vi "Calib_General_Setup.vi"(0 "Reference instrument":T3={"high limit (10V)"=4.0, "low limit (-10V)"=0.0, "Ch No"=4, "Off ch no"=0, "Calib filename"=path "", "Ref Instrument type"=enum."Enter Value"} {"Off ch no" min=0 max=1; "Ch No" min=0 max=7; "low limit (-10V)" min=-10 max=10 format="%.3f"; "high limit (10V)" min=-10 max=10 format="%.3f"}, 1 "Requested No of samples":i32=128 min=0 step=1, 2 "Sampling rate (Hz)":sgl=1000.0 format="%.2f", 5 "2nd ref instrument":T2={"2nd Ref type"=enum."LDA", "2nd inst present"=TRUE}, 9 "Temp":dbl=20.0 format="%.1f", 12 "Abs Press (mbar)":dbl=1005.0 format="%.2f") -> (8 "Output string":string, 10 "LDA Data":bool)   [LabVIEW 2017]
uses:
  Controls/Ref_Inst_type.ctl
  Controls/Graph_Type.ctl
  Globals/Meas_global.vi
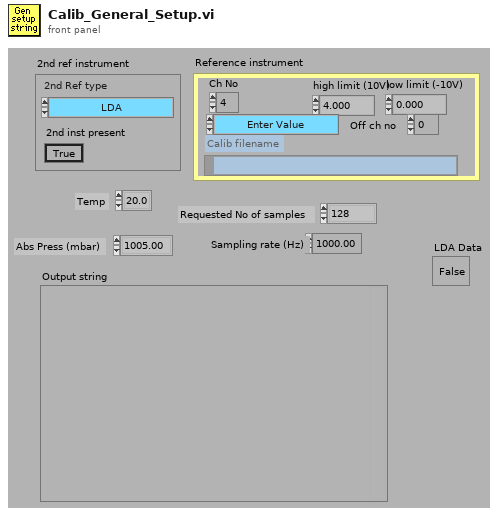
[diagram p1: front panel]
types:
  T1 = typedef "Ref_Inst_type.ctl" = enum16{"Propellor anemometer", "Pressure Transducer", "Raw voltage", "Pitot-static tube", "Preston tube", "Generic Linear", "Generic Polynomial", "Thermocouple", "LDA", "Enter Value", "ADAM Channel"}
  T2 = cluster{"2nd Ref type":T1, "2nd inst present":bool}
  T3 = cluster{"high limit (10V)":sgl, "low limit (-10V)":sgl, "Ch No":i16, "Off ch no":i8, "Calib filename":path, "Ref Instrument type":T1}
  T4 = typedef "Graph_Type.ctl" = enum16{"Show no graph", "Voltage trace", "Velocity trace", "Vel histogram", "Spectrum", "f.E(f) v Log f", "Auto-Corr"}
  T5 = cluster{"Plot 1":u16, "Plot 2":u16, "Save graph":u16, "Plot Type":T4}
  T6 = enum16{"From String to Cluster", "From Cluster to String"}
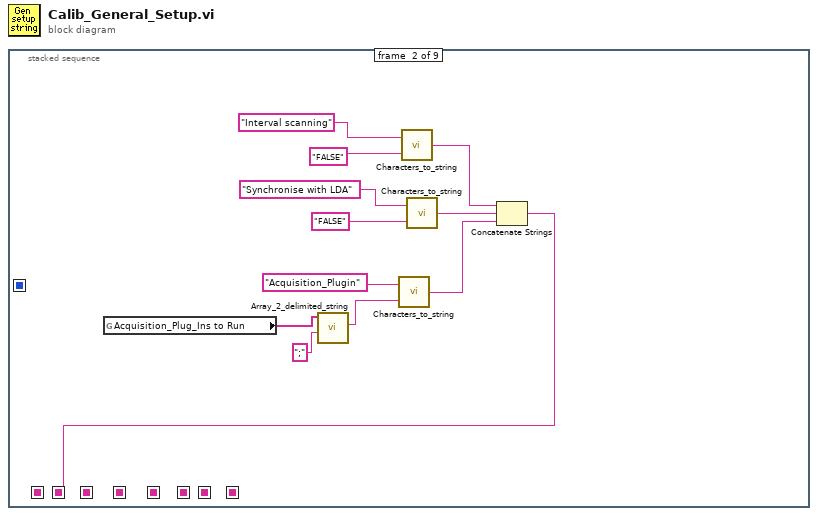
[diagram p0: block diagram]
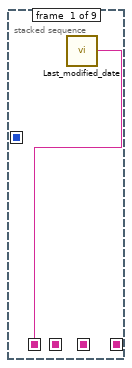
[diagram p2: hidden frame]
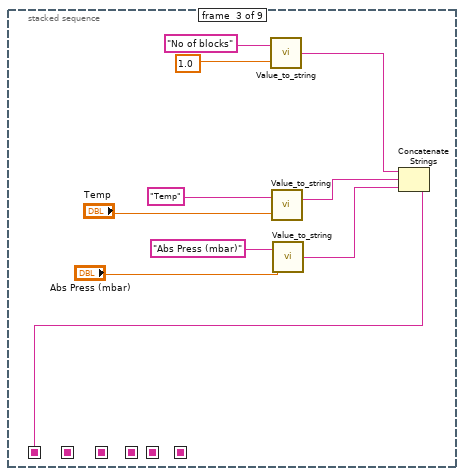
[diagram p3: hidden frame]
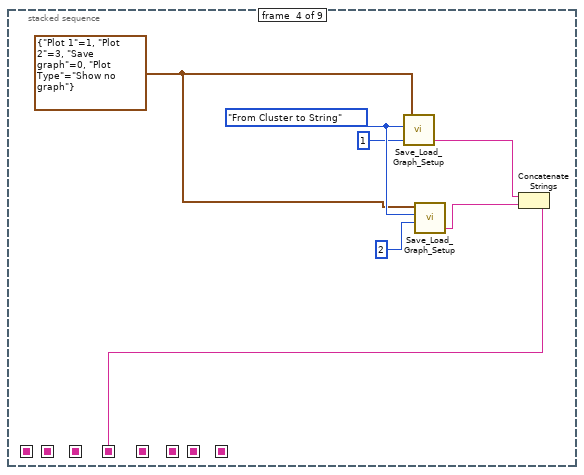
[diagram p4: hidden frame]
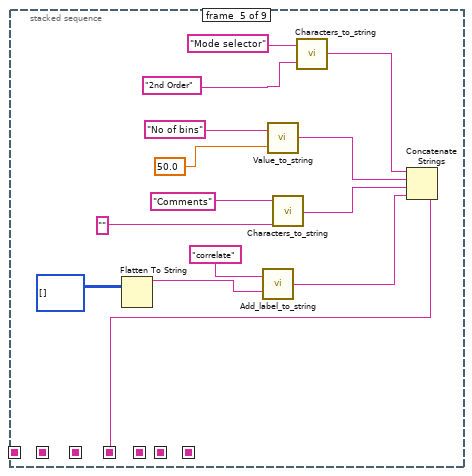
[diagram p5: hidden frame]
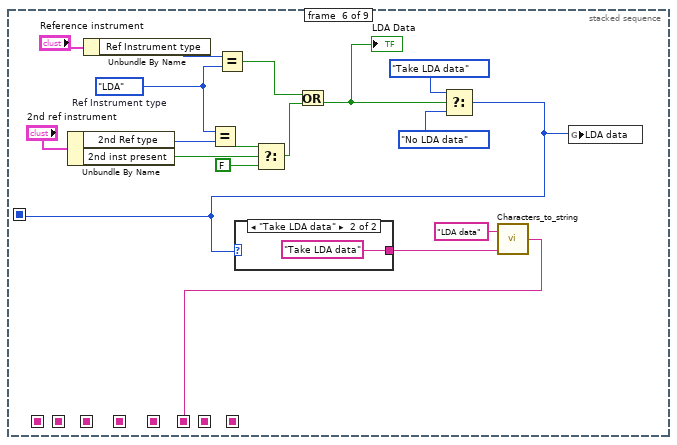
[diagram p6: hidden frame]
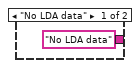
[diagram p7: hidden frame]
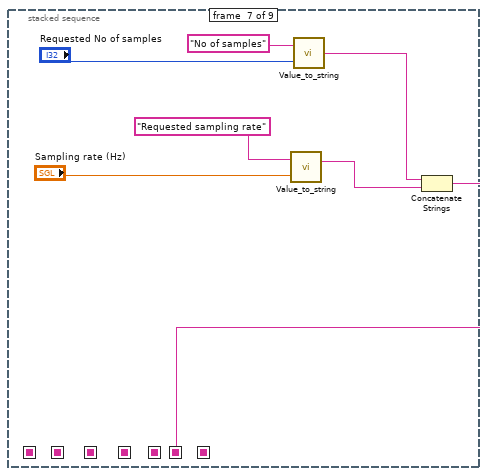
[diagram p8: hidden frame]
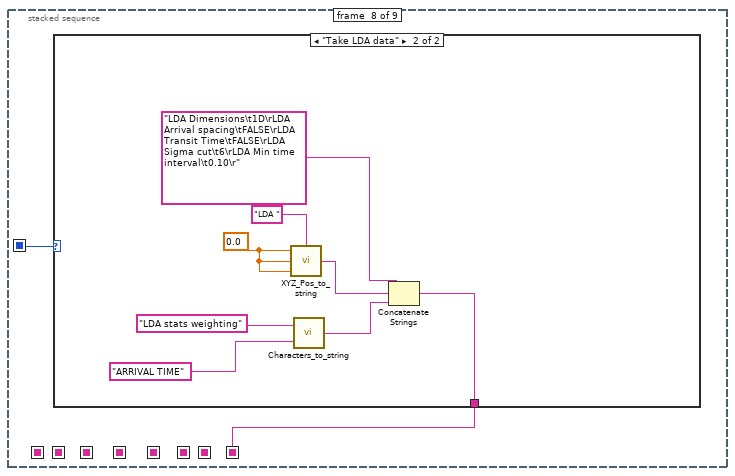
[diagram p9: hidden frame]
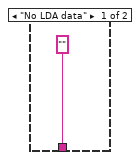
[diagram p10: hidden frame]
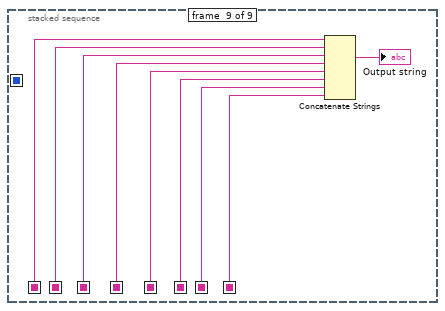
[diagram p11: hidden frame]
diagram:
  n1 = stacked-sequence {
    seq-local: [_ _ w22 _ _ _ _ _ _] -> [_ _ _ _ _ _ _ _ w90]
    seq-local: [_ w9 _ _ _ _ _ _ _] -> [_ _ _ _ _ _ _ _ w89]
    seq-local: [_ _ _ _ _ w59 _ _ _] -> [_ _ _ _ _ _ _ _ w85]
    seq-local: [_ _ _ _ _ _ w69 _ _] -> [_ _ _ _ _ _ _ _ w84]
    seq-local: [_ _ _ w25 _ _ _ _ _] -> [_ _ _ _ _ _ _ _ w87]
    seq-local: [_ _ _ _ w35 _ _ _ _] -> [_ _ _ _ _ _ _ _ w86]
    seq-local: [w1 _ _ _ _ _ _ _ _] -> [_ _ _ _ _ _ _ _ w83]
    seq-local: [_ _ _ _ _ w46 _ _ _] -> [_ _ _ _ _ _ _ w72 _]
    seq-local: [_ _ _ _ _ _ _ w71 _] -> [_ _ _ _ _ _ _ _ w82]
    frame #0 {
      n2 = call "Last_modified_date.vi"() -> ("RevisionString"=w1:string)  [unwired: 1 in, 1 out]
    }
    frame #1 {
      n3 = global read "Meas_global.vi" "Acquisition_Plug_Ins to Run"() -> (w4:string[])
      n4 = call "Array_2_delimited_string.vi"("delimiter (Tab)"=";", "Array of Strings"=w4) -> ("delimited string"=w3:string)  [unwired: 9 in]
      n5 = call "Characters_to_string.vi"("Characters to write"=w3, "Label for characters"="Acquisition_Plugin") -> ("Output string"=w5:string)
      n6 = call "Characters_to_string.vi"("Characters to write"="FALSE", "Label for characters"="Interval scanning") -> ("Output string"=w11:string)
      n7 = call "Characters_to_string.vi"("Characters to write"="FALSE", "Label for characters"="Synchronise with LDA") -> ("Output string"=w10:string)
      n8 = Concatenate Strings(w11, w10, w5) -> (w9:string)
    }
    frame #2 {
      n9 = call "Value_to_string.vi"("Value"=1.0, "Label for value"="No of blocks") -> ("Output string"=w16:string)  [unwired: 1 in]
      n10 = call "Value_to_string.vi"("Value"="Temp", "Label for value"="Temp") -> ("Output string"=w19:string)  [unwired: 1 in]
      n11 = call "Value_to_string.vi"("Value"="Abs Press (mbar)", "Label for value"="Abs Press (mbar)") -> ("Output string"=w18:string)  [unwired: 1 in]
      n12 = Concatenate Strings(w16, w19, w18) -> (w22:string)
    }
    frame #3 {
      w24 = T5 {"Plot 1"=1, "Plot 2"=3, "Save graph"=0, "Plot Type"=enum."Show no graph"} ("Graph in")
      w28 = T6."From Cluster to String" ("Mode")
      n13 = call "Save_Load_Graph_Setup.vi"("Graph Number"=1, "Mode"=w28, "Graph in"=w24) -> ("Setup String Out"=w30:string)  [unwired: 1 in, 2 out]
      n14 = call "Save_Load_Graph_Setup.vi"("Graph Number"=2, "Mode"=w28, "Graph in"=w24) -> ("Setup String Out"=w29:string)  [unwired: 1 in, 2 out]
      n15 = Concatenate Strings(w30, w29) -> (w25:string)
    }
    frame #4 {
      n16 = Flatten To String(anything=i8[][] [] ("correlate")) -> (data string=w31:string)  [unwired: 1 in, 4 out]
      n17 = call "Add_label_to_string.vi"("String to write"=w31, "File Label"="correlate") -> ("Output string"=w36:string)
      n18 = call "Value_to_string.vi"("Value"=50.0 ("Bins"), "Label for value"="No of bins") -> ("Output string"=w43:string)  [unwired: 1 in]
      n19 = call "Characters_to_string.vi"("Characters to write"="" ("Comments"), "Label for characters"="Comments") -> ("Output string"=w38:string)
      n20 = call "Characters_to_string.vi"("Characters to write"="2nd Order", "Label for characters"="Mode selector") -> ("Output string"=w40:string)
      n21 = Concatenate Strings(w40, w43, w38, w36) -> (w35:string)
    }
    frame #5 {
      w45 = Ref_Inst_type."LDA"  # Ref Instrument type
      n22 = Unbundle By Name("2nd ref instrument") -> ("2nd Ref type"=w54:T1, "2nd inst present"=w55:bool)
      n23 = Unbundle By Name("Reference instrument") -> ("Ref Instrument type"=w56:T1)
      n24 = Equal?(x=w45, y=w54) -> (x = y?=w53:bool)
      n25 = Equal?(x=w56, y=w45) -> (x = y?=w50:bool)
      n26 = Select(t=w53, s=w55, f=FALSE) -> (s? t:f=w51:bool)
      n27 = Or(x=w50, y=w51) -> (x .or. y?=w47:bool)
      "LDA Data" <- w47
      n28 = Select(t=enum16{"No LDA data", "Take LDA data"}."Take LDA data" ("LDA data"), s=w47, f=enum16{"No LDA data", "Take LDA data"}."No LDA data" ("LDA data")) -> (s? t:f=w46:enum16{"No LDA data", "Take LDA data"})
      n29 = case shown="\"Take LDA data\"" w46 {
        tunnel: ["No LDA data" "Take LDA data"] -> w60
        frame "No LDA data" {
        }
        frame "Take LDA data" {
        }
      }
      n30 = call "Characters_to_string.vi"("Characters to write"=w60, "Label for characters"="LDA data") -> ("Output string"=w59:string)
      n31 = global write "Meas_global.vi" "LDA data"(w46) -> ()
    }
    frame #6 {
      n32 = call "Value_to_string.vi"("Value"="Sampling rate (Hz)", "Label for value"="Requested sampling rate") -> ("Output string"=w67:string)  [unwired: 1 in]
      n33 = call "Value_to_string.vi"("Value"="Requested No of samples", "Label for value"="No of samples") -> ("Output string"=w68:string)  [unwired: 1 in]
      n34 = Concatenate Strings(w68, w67) -> (w69:string)
    }
    frame #7 {
      n35 = case shown="\"Take LDA data\"" w72 {
        tunnel: ["" w75] -> w71
        frame "No LDA data" {
        }
        frame "Take LDA data" {
          w81 = 0.0 ("X")
          n36 = call "XYZ_Pos_to_string.vi"("Position label"="LDA ", "Z"=w81, "Y"=w81, "X"=w81) -> ("Output string"=w77:string)
          n37 = call "Characters_to_string.vi"("Characters to write"="ARRIVAL TIME" ("LDA stats type"), "Label for characters"="LDA stats weighting") -> ("Output string"=w76:string)
          n38 = Concatenate Strings("LDA Dimensions\t1D\rLDA Arrival spacing\tFALSE\rLDA Transit Time\tFALSE\rLDA Sigma cut\t6\rLDA Min time interval\t0.10\r" ("String"), w77, w76) -> (w75:string)
        }
      }
    }
    frame #8 {
      n39 = Concatenate Strings(w83, w89, w90, w87, w86, w85, w84, w82) -> (→"Output string":string)
    }
  }
